vi "String_to_move_stage.vi"(0 "reference IN":refnum<k7>, 5 "Movement string":string, 7 "XY step size (µm)":dbl, 9 "Z step size (µm)":dbl, 11 "error in (no error)":errorcluster) -> (4 "reference OUT":refnum<k7>, 6 "String":string, 15 "error OUT":errorcluster)   [LabVIEW 2020]
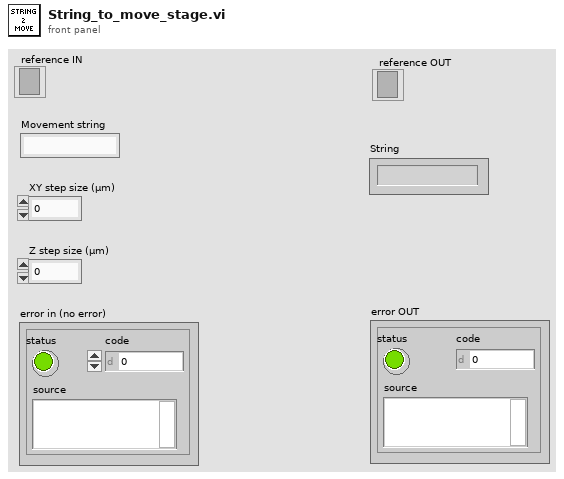
[diagram p1: front panel]
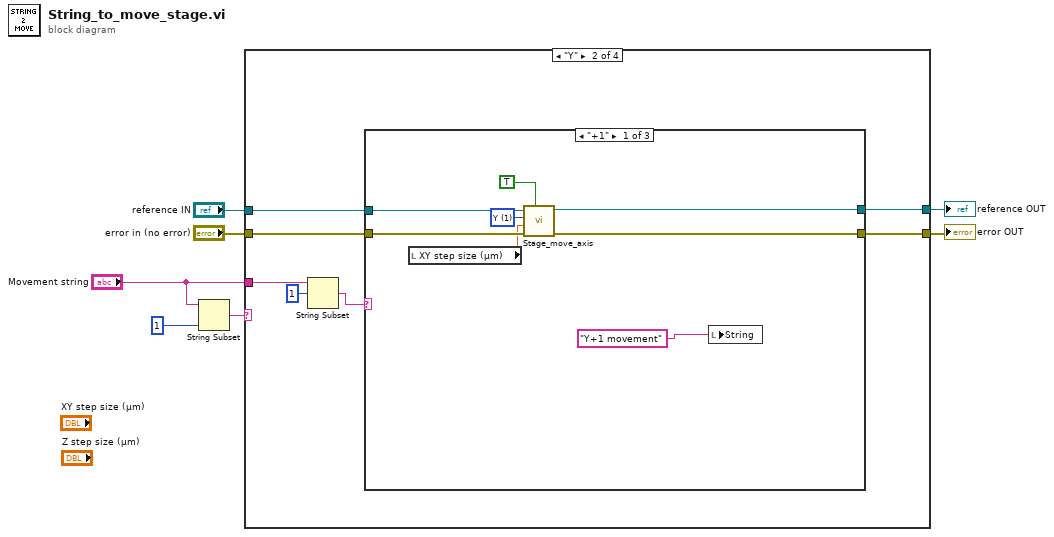
[diagram p0: block diagram]
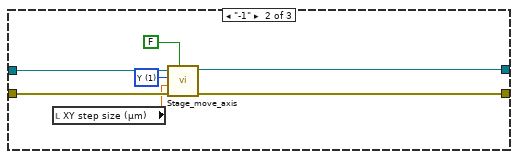
[diagram p3: hidden frame]
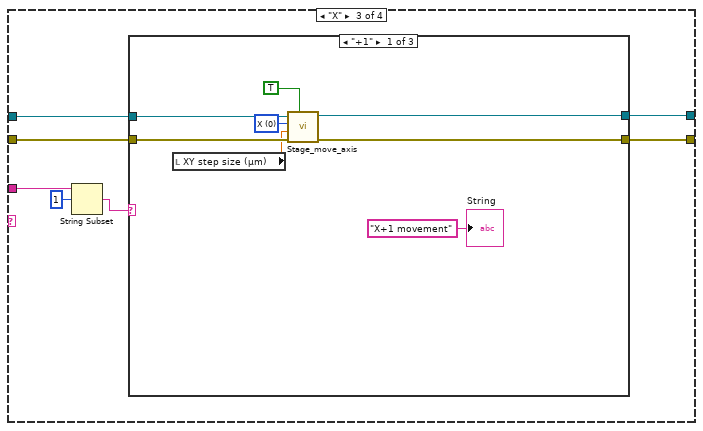
[diagram p5: hidden frame]
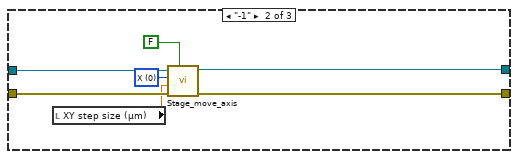
[diagram p6: hidden frame]
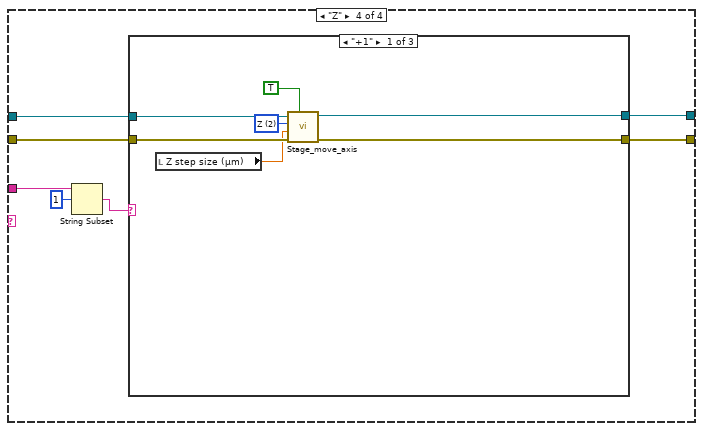
[diagram p8: hidden frame]
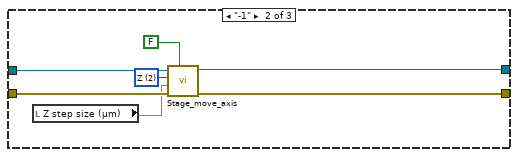
[diagram p9: hidden frame]
diagram:
  n1 = String Subset(string="Movement string", length (rest)=1 ("length (rest)")) -> (substring=w7:string)  [unwired: 1 in]
  n2 = case shown="\"Y\"" w7 {
    tunnel: "Movement string" -> [_ w16 w40 w64]
    tunnel: "reference IN" -> [w9 w13 w37 w61]
    tunnel: "error in (no error)" -> [w8 w12 w36 w60]
    tunnel: [w9 w11 w35 w59] -> w3
    tunnel: [w8 w10 w34 w58] -> w2
    frame "False", Default {
    }
    frame "Y" {
      n3 = String Subset(string=w16, offset (0)=1) -> (substring=w14:string)  [unwired: 1 in]
      n4 = case shown="\"+1\"" w14 {
        tunnel: w13 -> [w24 w31 w33]
        tunnel: w12 -> [w23 w30 w32]
        tunnel: [w19 w26 w33] -> w11
        tunnel: [w18 w25 w32] -> w10
        frame "+1" {
          w22 = u16 1 items=["X", "Y", "Z"] ("Axes Select")
          n5 = local read "XY step size (µm)"() -> (w20:dbl)
          n6 = call "Stage_move_axis.vi"("Direction true means positive increment"=TRUE, "error in (no error)"=w23, "Distance micrometer"=w20, "Axes Select"=w22, "reference IN"=w24) -> ("error OUT"=w18:errorcluster, "reference OUT"=w19:refnum<k7>)  [unwired: 5 in]
          n7 = local write "String"("Y+1 movement" ("String")) -> ()
        }
        frame "-1" {
          w29 = u16 1 items=["X", "Y", "Z"] ("Axes Select")
          n8 = local read "XY step size (µm)"() -> (w27:dbl)
          n9 = call "Stage_move_axis.vi"("Direction true means positive increment"=FALSE, "error in (no error)"=w30, "Distance micrometer"=w27, "Axes Select"=w29, "reference IN"=w31) -> ("error OUT"=w25:errorcluster, "reference OUT"=w26:refnum<k7>)  [unwired: 5 in]
        }
        frame Default {
        }
      }
    }
    frame "X" {
      n10 = String Subset(string=w40, offset (0)=1) -> (substring=w38:string)  [unwired: 1 in]
      n11 = case shown="\"+1\"" w38 {
        tunnel: w37 -> [w48 w55 w57]
        tunnel: w36 -> [w47 w54 w56]
        tunnel: [w43 w50 w57] -> w35
        tunnel: [w42 w49 w56] -> w34
        frame "+1" {
          w46 = u16 0 items=["X", "Y", "Z"] ("Axes Select")
          n12 = local read "XY step size (µm)"() -> (w44:dbl)
          n13 = call "Stage_move_axis.vi"("Direction true means positive increment"=TRUE, "error in (no error)"=w47, "Distance micrometer"=w44, "Axes Select"=w46, "reference IN"=w48) -> ("error OUT"=w42:errorcluster, "reference OUT"=w43:refnum<k7>)  [unwired: 5 in]
          "String" <- "X+1 movement" ("String")
        }
        frame "-1" {
          w53 = u16 0 items=["X", "Y", "Z"] ("Axes Select")
          n14 = local read "XY step size (µm)"() -> (w51:dbl)
          n15 = call "Stage_move_axis.vi"("Direction true means positive increment"=FALSE, "error in (no error)"=w54, "Distance micrometer"=w51, "Axes Select"=w53, "reference IN"=w55) -> ("error OUT"=w49:errorcluster, "reference OUT"=w50:refnum<k7>)  [unwired: 5 in]
        }
        frame Default {
        }
      }
    }
    frame "Z" {
      n16 = String Subset(string=w64, offset (0)=1) -> (substring=w62:string)  [unwired: 1 in]
      n17 = case shown="\"+1\"" w62 {
        tunnel: w61 -> [w71 w78 w80]
        tunnel: w60 -> [w70 w77 w79]
        tunnel: [w67 w74 w80] -> w59
        tunnel: [w66 w73 w79] -> w58
        frame "+1" {
          w69 = u16 2 items=["X", "Y", "Z"] ("Axes Select")
          n18 = local read "Z step size (µm)"() -> (w65:dbl)
          n19 = call "Stage_move_axis.vi"("Direction true means positive increment"=TRUE, "error in (no error)"=w70, "Distance micrometer"=w65, "Axes Select"=w69, "reference IN"=w71) -> ("error OUT"=w66:errorcluster, "reference OUT"=w67:refnum<k7>)  [unwired: 5 in]
        }
        frame "-1" {
          w76 = u16 2 items=["X", "Y", "Z"] ("Axes Select")
          n20 = local read "Z step size (µm)"() -> (w72:dbl)
          n21 = call "Stage_move_axis.vi"("Direction true means positive increment"=FALSE, "error in (no error)"=w77, "Distance micrometer"=w72, "Axes Select"=w76, "reference IN"=w78) -> ("error OUT"=w73:errorcluster, "reference OUT"=w74:refnum<k7>)  [unwired: 5 in]
        }
        frame Default {
        }
      }
    }
  }
  "reference OUT" <- w3
  "error OUT" <- w2
